vi "ReadProperties.vi"(10 "Thing":string="Thing") -> (3 "All":string[][](array[string]))   [LabVIEW 2020]
panel:
  out "value":T1
  out "Comm":T2
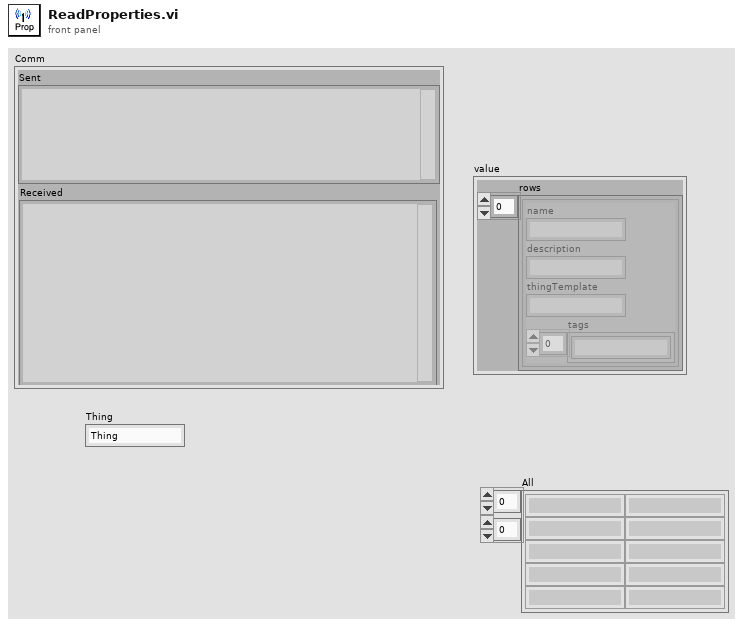
[diagram p1: front panel]
types:
  T1 = cluster{"rows":cluster{"name":string, "description":string, "thingTemplate":string, "tags":string[]}[]}
  T2 = cluster{"url":string, "sent headers":string, "sent body":string, "headers":string, "body":string, "Sent":string, "Received":string}
  T3 = cluster{"Name":string, "BaseURL":string, "AppKey":string, "Headers":string[], "Timeout":i32}
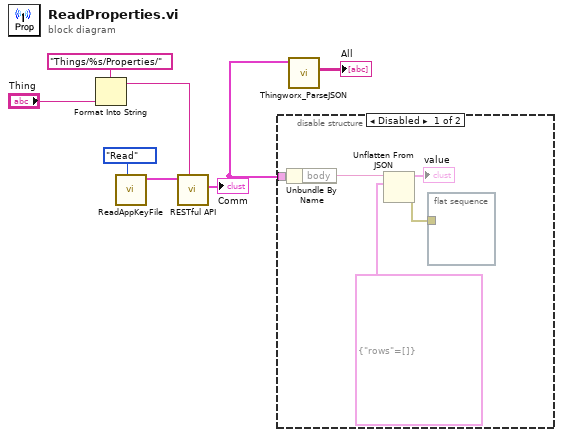
[diagram p0: block diagram]
diagram:
  n1 = Format Into String(format string="Things/%s/Properties/" ("url"), "Thing") -> (resulting string=w3:string)  [unwired: 2 in, 1 out]
  n2 = call "ReadAppKeyFile.vi"("Task"=enum16{"Read", "Write"}."Read") -> ("Device Out"=w7:T3)  [unwired: 8 in, 2 out]
  n3 = call "RESTful API.vi"("url"=w3, "Device In"=w7) -> ("Comm"=w2:T2)  [unwired: 7 in, 2 out]
  "Comm" <- w2
  n4 = disable-structure shown="Disabled" {
    disable-tunnel: w2 -> [w9 _]
    frame Disabled {
      n5 = Unbundle By Name(w9) -> ("body"=w10:string)
      n6 = Unflatten From JSON(JSON string=w10, type and defaults=T1 {"rows"=[]} ("Cluster")) -> (value=→"value":T1, error out=w8:errorcluster)  [unwired: 5 in]
      n7 = flat-sequence {
        tunnel: w8 -> [_]
        frame #0 {
        }
      }
    }
    frame Enabled {
    }
  }
  n8 = call "Thingworx_ParseJSON.vi"("Comm"=w2) -> ("Table Control"=→"All":string[][])  [unwired: 9 in, 1 out]
